vi "Test WebSockets Connection.vi"() -> ()   [LabVIEW 2013]
uses:
  <vilib>/LabVIEW Open Source Project/MQTT Connection/MQTT_Connection/Connection/Connection.lvclass
  <vilib>/LabVIEW Open Source Project/MQTT Websockets Connection/MQTT_Websockets/Connection/WebsocketsConnection.lvclass
panel:
  out "server session error 2":errorcluster
  out "Bytes 2":u8[](array[numeric]) format="%08b"
  out "client session error 2":errorcluster
  out "value 2":dbl
  out "value":dbl
  out "listener error":errorcluster
  out "client session error":errorcluster
  out "server session error":errorcluster
  out "Bytes":u8[](array[numeric]) format="%08b"
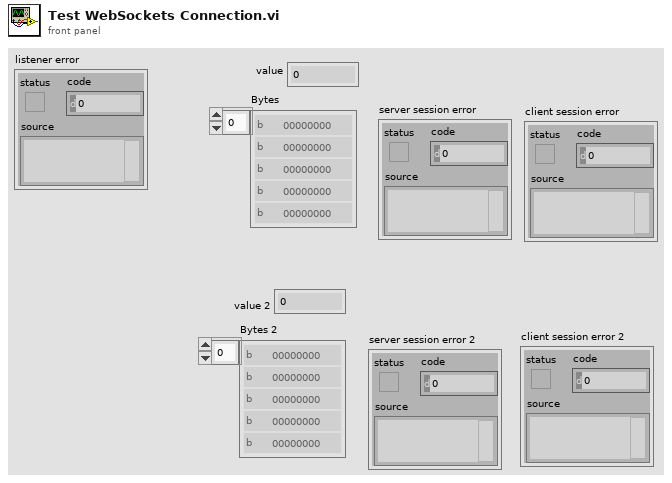
[diagram p1: front panel]
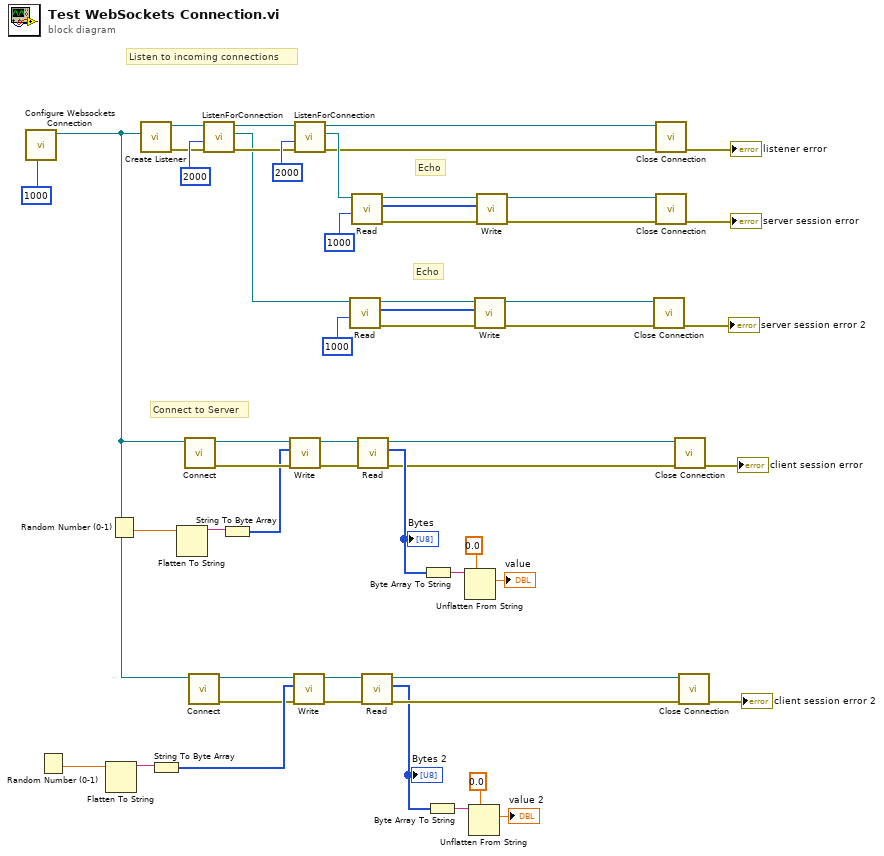
[diagram p0: block diagram]
diagram:
  # "Echo"
  # "Connect to Server"
  # "Echo"
  # "Listen to incoming connections"
  n1 = call <vilib>:"Configure Websockets Connection.vi"("timeout (5000 ms)"=1000 ("timeout (100ms)")) -> ("WSConnection"=w15:refnum<class "WebsocketsConnection.lvclass">)  [unwired: 9 in, 1 out]
  n2 = Random Number (0-1)() -> (number: 0 to 1=w20:dbl)
  n3 = Flatten To String(anything=w20) -> (data string=w21:string)  [unwired: 3 in, 2 out]
  n4 = Random Number (0-1)() -> (number: 0 to 1=w42:dbl)
  n5 = call <vilib>:"Create Listener.vi"("Connection Configuration"=w15) -> ("error out"=w6:errorcluster, "Listener"=w8:refnum<class "Connection.lvclass">)  [unwired: 9 in]
  n6 = String To Byte Array(string=w21) -> (unsigned byte array=w22:u8[])
  n7 = Flatten To String(anything=w42) -> (data string=w41:string)  [unwired: 3 in, 2 out]
  n8 = call <vilib>:"Connect.vi"("Connection in"=w15) -> ("error out"=w45:errorcluster, "Connection out"=w49:refnum<class "WebsocketsConnection.lvclass">)  [unwired: 9 in]
  n9 = call <vilib>:"Connect.vi"("Connection in"=w15) -> ("error out"=w19:errorcluster, "Connection out"=w16:refnum<class "WebsocketsConnection.lvclass">)  [unwired: 9 in]
  n10 = call <vilib>:"ListenForConnection.vi"("error in (no error)"=w6, "timeout (2000 ms)"=2000 ("bytes to read (100)"), "Listener"=w8) -> ("error out"=w5:errorcluster, "Connection"=w4:refnum<class "Connection.lvclass">, "Listener out"=w7:refnum<class "Connection.lvclass">)  [unwired: 5 in, 1 out]
  n11 = String To Byte Array(string=w41) -> (unsigned byte array=w40:u8[])
  n12 = call <vilib>:"Write.vi"("error in (no error)"=w45, "Bytes"=w40, "Connection in"=w49) -> ("error out"=w46:errorcluster, "Connection"=w48:refnum<class "WebsocketsConnection.lvclass">)  [unwired: 7 in]
  n13 = call <vilib>:"Write.vi"("error in (no error)"=w19, "Bytes"=w22, "Connection in"=w16) -> ("error out"=w18:errorcluster, "Connection"=w17:refnum<class "WebsocketsConnection.lvclass">)  [unwired: 7 in]
  n14 = call <vilib>:"ListenForConnection.vi"("error in (no error)"=w5, "timeout (2000 ms)"=2000 ("bytes to read (100)"), "Listener"=w7) -> ("error out"=w34:errorcluster, "Connection"=w52:refnum<class "Connection.lvclass">, "Listener out"=w54:refnum<class "Connection.lvclass">)  [unwired: 5 in, 1 out]
  n15 = call <vilib>:"Read.vi"("timeout (5000 ms)"=1000 ("bytes to read (100)"), "TCPConnection in"=w4) -> ("error out"=w13:errorcluster, "Bytes"=w12:u8[], "TCPConnection out"=w11:refnum<class "Connection.lvclass">)  [unwired: 5 in, 2 out]
  n16 = call <vilib>:"Read.vi"("timeout (5000 ms)"=1000 ("bytes to read (100)"), "TCPConnection in"=w52) -> ("error out"=w47:errorcluster, "Bytes"=w50:u8[], "TCPConnection out"=w51:refnum<class "Connection.lvclass">)  [unwired: 5 in, 2 out]
  n17 = call <vilib>:"Read.vi"("error in (no error)"=w46, "TCPConnection in"=w48) -> ("error out"=w2:errorcluster, "Bytes"=w39:u8[], "TCPConnection out"=w31:refnum<class "WebsocketsConnection.lvclass">)  [unwired: 5 in, 2 out]
  "Bytes" <- w39
  n18 = call <vilib>:"Read.vi"("error in (no error)"=w18, "TCPConnection in"=w17) -> ("error out"=w28:errorcluster, "Bytes"=w23:u8[], "TCPConnection out"=w29:refnum<class "WebsocketsConnection.lvclass">)  [unwired: 5 in, 2 out]
  "Bytes 2" <- w23
  n19 = Byte Array To String(unsigned byte array=w39) -> (string=w38:string)
  n20 = Byte Array To String(unsigned byte array=w23) -> (string=w24:string)
  n21 = Unflatten From String(type=0.0, binary string=w38) -> (value=→"value":dbl)  [unwired: 3 in, 2 out]
  n22 = Unflatten From String(type=0.0, binary string=w24) -> (value=→"value 2":dbl)  [unwired: 3 in, 2 out]
  n23 = call <vilib>:"Write.vi"("error in (no error)"=w13, "Bytes"=w12, "Connection in"=w11) -> ("error out"=w14:errorcluster, "Connection"=w1:refnum<class "Connection.lvclass">)  [unwired: 7 in]
  n24 = call <vilib>:"Write.vi"("error in (no error)"=w47, "Bytes"=w50, "Connection in"=w51) -> ("error out"=w32:errorcluster, "Connection"=w43:refnum<class "Connection.lvclass">)  [unwired: 7 in]
  n25 = call <vilib>:"Close Connection.vi"("error in (no error)"=w14, "Connection in"=w1) -> ("error out"=→"server session error 2":errorcluster)  [unwired: 8 in, 1 out]
  n26 = call <vilib>:"Close Connection.vi"("error in (no error)"=w34, "Connection in"=w54) -> ("error out"=→"listener error":errorcluster)  [unwired: 8 in, 1 out]
  n27 = call <vilib>:"Close Connection.vi"("error in (no error)"=w32, "Connection in"=w43) -> ("error out"=→"server session error":errorcluster)  [unwired: 8 in, 1 out]
  n28 = call <vilib>:"Close Connection.vi"("error in (no error)"=w2, "Connection in"=w31) -> ("error out"=→"client session error":errorcluster)  [unwired: 8 in, 1 out]
  n29 = call <vilib>:"Close Connection.vi"("error in (no error)"=w28, "Connection in"=w29) -> ("error out"=→"client session error 2":errorcluster)  [unwired: 8 in, 1 out]
